vi "Panel.vi"(11 "Terminal in":refnum<class "Terminal.lvclass">) -> ()   [LabVIEW 2020, in "Terminal.lvlib" / "Terminal.lvclass"]
uses:
  Terminal.lvclass
  C:/Program Files (x86)/National Instruments/LabVIEW 2020/vi.lib/IlluminatedG/IG OOPanel/OOPanel/Panel/Panel.lvclass
  <vilib>/IlluminatedG/IG OOPanel/OOPanel/Panel/Basic UI State.ctl
  Terminal.lvclass/Terminal.ctl
  Key Event Data.ctl
  <vilib>/event_ctls.llb/eventvkey.ctl
  <vilib>/IlluminatedG/IG OOPanel/OOPanel/Panel/Panel.lvclass
  <vilib>/IlluminatedG/IG OOPanel/OOPanel/OOPanel.lvlib
  Terminal.lvlib
  C:/dev/IlluminatedG/lv-stream-terminal/Terminal/Terminal/Terminal.lvclass
panel:
  in  "Scrollbar":i32(c297)
  out "Overlay":picture
  out "Text":picture
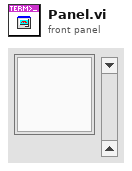
[diagram p1: front panel]
types:
  T1 = typedef "OOPanel.lvlib/Panel.lvclass/Basic UI State.ctl" = enum16{"Init", "Run", "Close"}
  T2 = typedef "Terminal.lvlib/Key Event Data.ctl" = cluster{"Char":i16, "VKey":T3, "ScanCode":i16, "Ctrl":bool}
  T3 = typedef "eventvkey.ctl" = enum16{"ASCII", "Enter", "Return", "Shift", "Ctrl", "Alt", "Cmd", "Opt", "Caps", "NumLock", "Clear", "Break", "Up", "Down", "Left", "Right", "Insert", "Delete", "Home", "End", "PageUp", "PageDown", "Escape", "Help", "Pause", "ScrollLock", "F1", "F2", "F3", "F4", "F5", "F6", "F7", "F8", "F9", "F10", "F11", "F12", "F13", "F14", "F15", "F16", "F17", "F18", "F19", "F20", "F21", "F22", "F23", "F24", "Play", "VolumeUp", "VolumeDown", "Mute", "Two Byte Char"}
  T4 = typedef "Terminal.lvlib/Terminal.lvclass/Incoming Events.ctl" = cluster{"Update":refnum<user-event>}
  T5 = typedef "OOPanel.lvlib/Panel.lvclass/Panel Events.ctl" = cluster{"Visbility":refnum<user-event>, "Close":refnum<user-event>}
  T6 = typedef "OOPanel.lvlib/Panel.lvclass/Visibility State.ctl" = enum16{"Idle", "Closed", "Hidden", "Visible", "Subpanel"}
  T7 = typedef "LVRectTypeDef.ctl" = cluster{"Left":i16, "Top":i16, "Right":i16, "Bottom":i16}
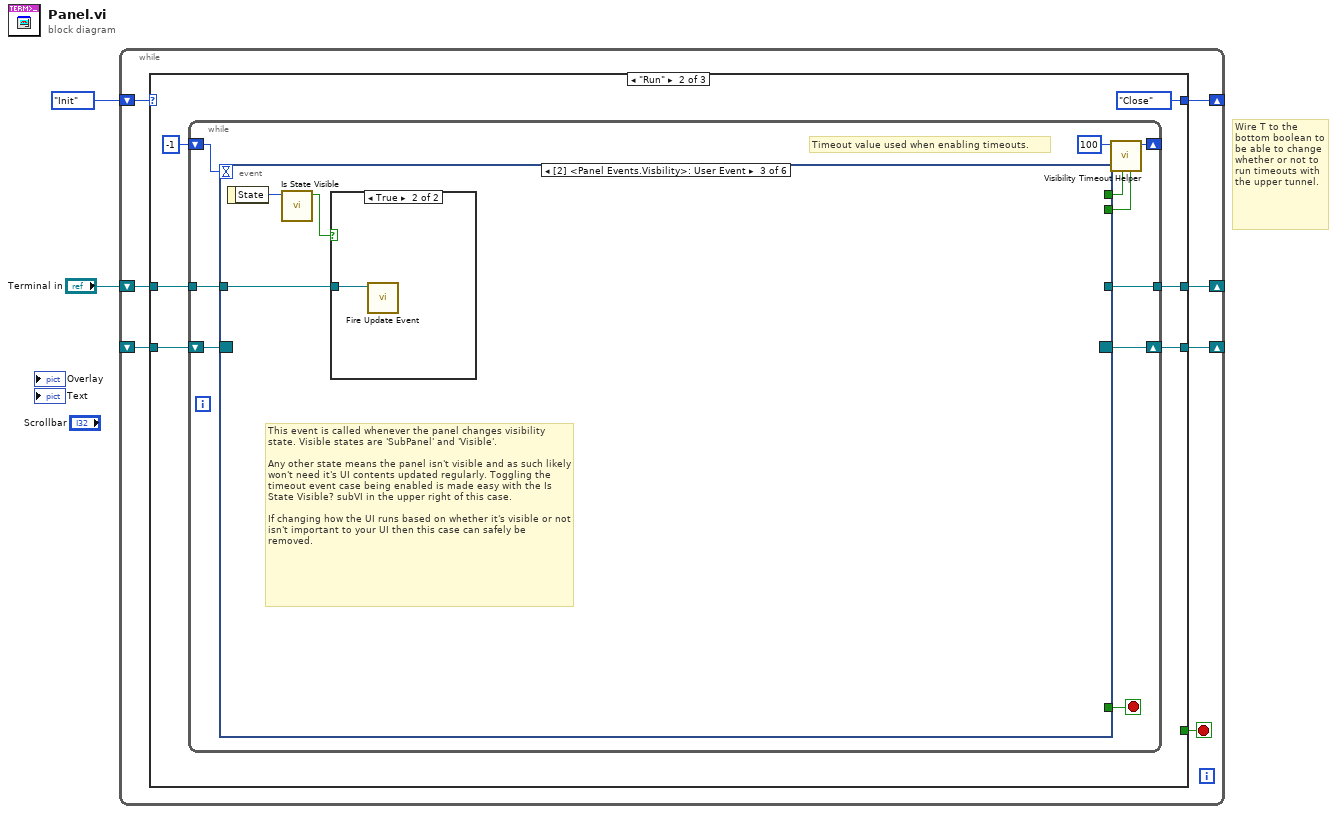
[diagram p0: block diagram]
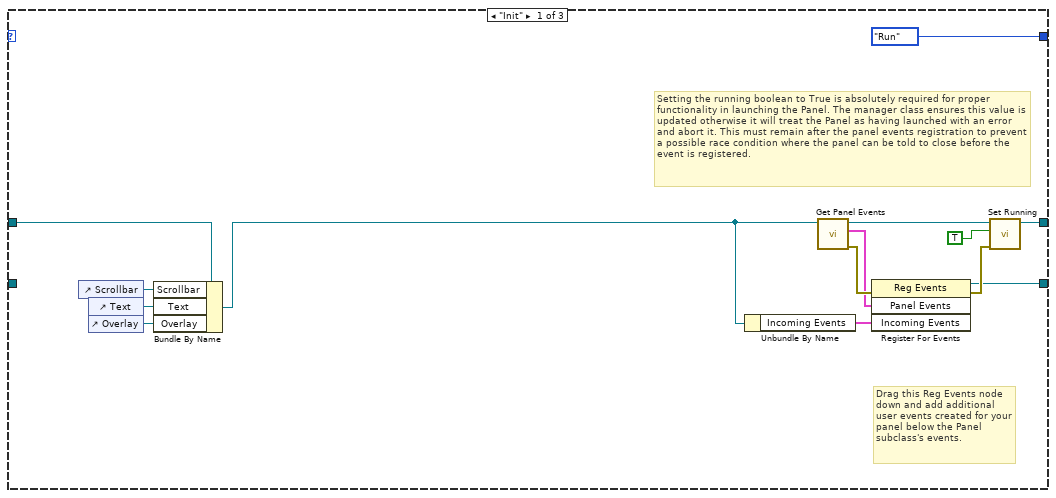
[diagram p2: hidden frame]
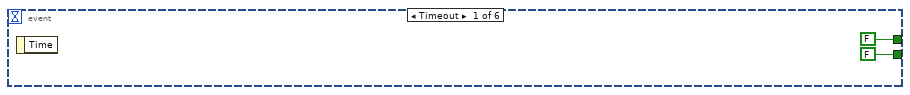
[diagram p3: hidden frame]
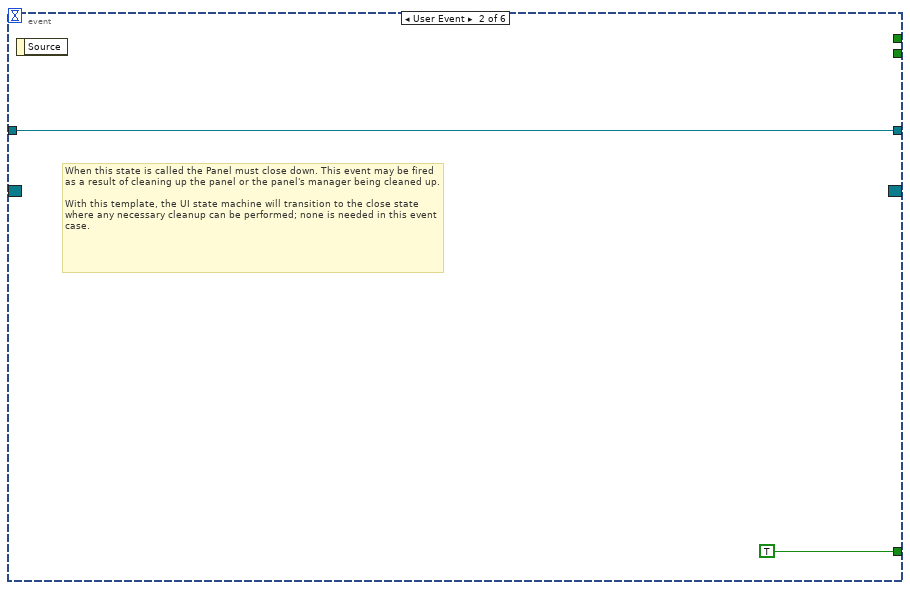
[diagram p4: hidden frame]
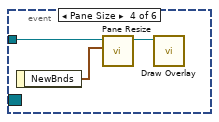
[diagram p6: hidden frame]
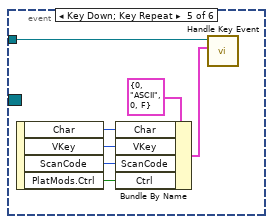
[diagram p7: hidden frame]
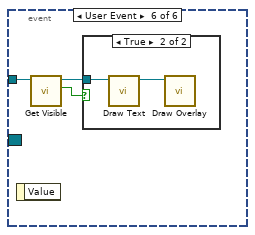
[diagram p8: hidden frame]
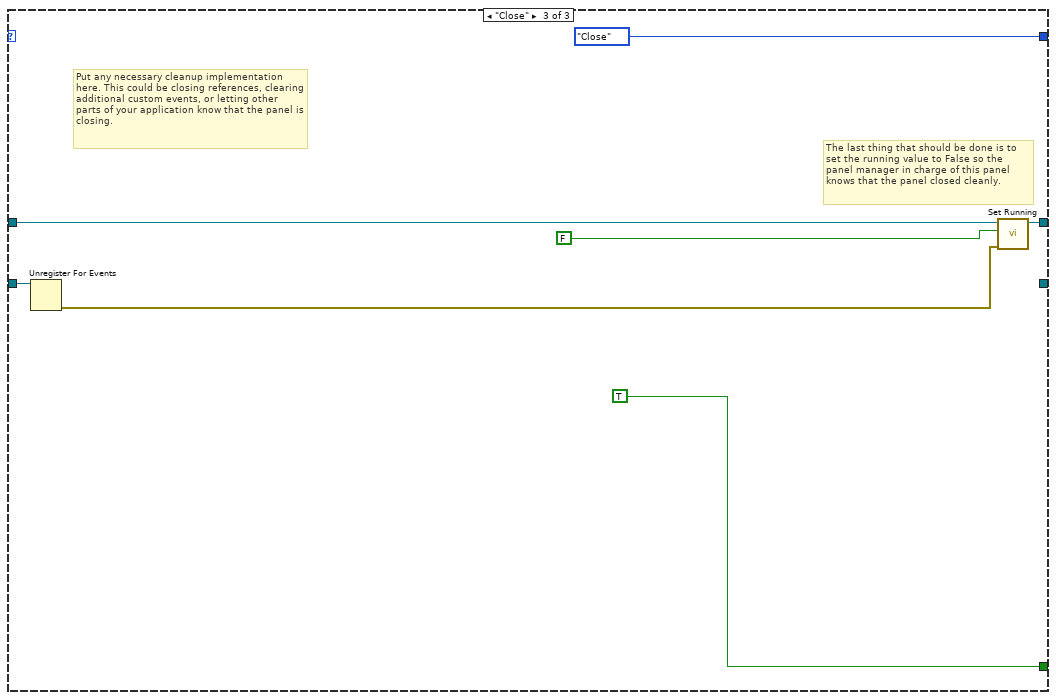
[diagram p10: hidden frame]
diagram:
  # "Wire T to the bottom boolean to be able to change whether or not to run timeouts with the upper tunnel."
  n1 = while {
    shift-right: [w8] -> _
    shift-left: _ -> [w9]
    shift-right: [w6] -> _
    shift-left: Basic_UI_State."Init" ("Basic UI State") -> [w7]
    shift-right: [w4] -> _
    shift-left: "Terminal in" -> [w3]
    stop <- w5 stop-if-true
    n2 = case shown="\"Run\"" w7 {
      tunnel: w9 -> [_ w29 w65]
      tunnel: [w17 w27 _] -> w8
      tunnel: [Basic_UI_State."Run" ("Basic UI State") Basic_UI_State."Close" ("Basic UI State") Basic_UI_State."Close" ("Basic UI State")] -> w6
      tunnel: [_ _ TRUE] -> w5
      tunnel: [w16 w24 w63] -> w4
      tunnel: w3 -> [w12 w25 w64]
      frame "Init" {
        # "Setting the running boolean to True is absolutely required for proper functionality in launching the Panel. The manager class ensures this value is updated otherwise it will treat the Panel as having launched with an error and abort it. This must remain after the panel events registration to prevent a possible race condition where the panel can be told to close before the event is registered."
        # "Drag this Reg Events node down and add additional user events created for your panel below the Panel subclass's events."
        n3 = control-ref of="Scrollbar"() -> (w15:refnum<vi>)
        n4 = control-ref of="Text"() -> (w14:refnum<vi>)
        n5 = control-ref of="Overlay"() -> (w13:refnum<vi>)
        n6 = Bundle By Name(cluster=w12, "Scrollbar"=w15, "Text"=w14, "Overlay"=w13) -> (w11:refnum<class "Terminal.lvclass">)
        n7 = Unbundle By Name(w11) -> ("Incoming Events"=w10:T4)
        n8 = call <vilib>:"Get Panel Events.vi"("Panel in"=w11) -> ("error out"=w23:errorcluster, "Panel Events"=w19:T5, "Panel out"=w20:refnum<class "Terminal.lvclass">)  [unwired: 8 in]
        n9 = register-events(error in=w23, w19, w10) -> (reference out=w17:refnum<event-registration>, error out=w21:errorcluster)  [unwired: 1 in]
        n10 = call <vilib>:"Set Running.vi"("error in (no error)"=w21, "Running"=TRUE, "Panel in"=w20) -> ("Panel out"=w16:refnum<class "Terminal.lvclass">)  [unwired: 7 in, 1 out]
      }
      frame "Run" {
        n11 = while {
          shift-right: [w35] -> w27
          shift-left: w29 -> [w36]
          shift-right: [w38] -> _
          shift-left: -1 ("Timeout") -> [w37]
          tunnel: w25 -> [w31]
          tunnel: [w30] -> w24
          stop <- w32 stop-if-true
          # "Timeout value used when enabling timeouts."
          n12 = event shown="[2] <Panel Events.Visbility>: User Event" {
            selector: w36 -> [_ _ _ _ _ _]
            dyn-events: [_ _ _ _ _ _] -> w35
            timeout: w37 -> [_ _ _ _ _ _]
            tunnel: [FALSE _ _ _ _ _] -> w34
            tunnel: [FALSE _ _ _ _ _] -> w33
            tunnel: [_ TRUE _ _ _ _] -> w32
            tunnel: w31 -> [_ w42 w44 w48 w52 w60]
            tunnel: [_ w42 _ _ _ _] -> w30
            event Timeout {
              n13 = event-data() -> ()  [unwired: 1 in, 1 out]
            }
            event User Event {
              # "When this state is called the Panel must close down. This event may be fired as a result of cleaning up the panel or the panel's manager being cleaned up.\n\nWith this template, the UI state machine will transition to the close state where any necessary cleanup can be performed; none is needed in this event case."
              n14 = event-data() -> ()  [unwired: 1 in, 1 out]
            }
            event User Event {
              # "This event is called whenever the panel changes visibility state. Visible states are 'SubPanel' and 'Visible'.\n\nAny other state means the panel isn't visible and as such likely won't need it's UI contents updated regularly. Toggling the timeout event case being enabled is made easy with the Is State Visible? subVI in the upper right of this case.\n\nIf changing how the UI runs based on whether it's visible or not isn't important to your UI then this case can safely be removed."
              n15 = event-data() -> ("State"=w46:T6)  [unwired: 1 in]
              n16 = call <vilib>:"Is State Visible.vi"("Visibility"=w46) -> ("Visible"=w45:bool)  [unwired: 10 in]
              n17 = case shown="True" w45 {
                tunnel: w44 -> [_ w47]
                frame False {
                }
                frame True {
                  n18 = call "Fire Update Event.vi"("Terminal in"=w47) -> ()  [unwired: 9 in, 2 out]
                }
              }
            }
            event Pane Size {
              n19 = event-data() -> ("NewBnds"=w50:T7)  [unwired: 1 in]
              n20 = call "Pane Resize.vi"("NewBnds"=w50, "Terminal in"=w48) -> ("Terminal out"=w49:refnum<class "Terminal.lvclass">)  [unwired: 8 in, 1 out]
              n21 = call "Draw Overlay.vi"("Terminal in"=w49) -> ()  [unwired: 9 in, 2 out]
            }
            event Key Down; Key Repeat {
              n22 = event-data() -> ("Char"=w56:i16, "VKey"=w55:T3, "ScanCode"=w54:i16, "PlatMods.Ctrl"=w53:bool)  [unwired: 1 in]
              n23 = Bundle By Name(cluster=T2 {"Char"=0, "VKey"=enum."ASCII", "ScanCode"=0, "Ctrl"=FALSE} ("Key Event Data"), "Char"=w56, "VKey"=w55, "ScanCode"=w54, "Ctrl"=w53) -> (w51:T2)
              n24 = call "Handle Key Event.vi"("Key Event Data"=w51, "Terminal in"=w52) -> ()  [unwired: 8 in, 2 out]
            }
            event User Event {
              n25 = event-data() -> ()  [unwired: 1 in, 1 out]
              n26 = call <vilib>:"Get Visible.vi"("Panel in"=w60) -> ("Visible"=w59:bool, "Panel out"=w58:refnum<class "Terminal.lvclass">)  [unwired: 8 in, 1 out]
              n27 = case shown="True" w59 {
                tunnel: w58 -> [_ w62]
                frame False {
                }
                frame True {
                  n28 = call "Draw Text.vi"("Terminal in"=w62) -> ("Terminal out"=w61:refnum<class "Terminal.lvclass">)  [unwired: 9 in, 1 out]
                  n29 = call "Draw Overlay.vi"("Terminal in"=w61) -> ()  [unwired: 9 in, 2 out]
                }
              }
            }
          }
          n30 = call <vilib>:"Visibility Timeout Helper.vi"("Update?"=w33, "Use Timeout?"=w34, "Visible Timeout mS"=100) -> ("Timeout"=w38:i32)  [unwired: 8 in]
        }
      }
      frame "Close" {
        # "Put any necessary cleanup implementation here. This could be closing references, clearing additional custom events, or letting other parts of your application know that the panel is closing."
        # "The last thing that should be done is to set the running value to False so the panel manager in charge of this panel knows that the panel closed cleanly."
        n31 = Unregister For Events(event registration refnum=w65) -> (error out=w67:errorcluster)  [unwired: 1 in]
        n32 = call <vilib>:"Set Running.vi"("error in (no error)"=w67, "Running"=FALSE, "Panel in"=w64) -> ("Panel out"=w63:refnum<class "Terminal.lvclass">)  [unwired: 7 in, 1 out]
      }
    }
  }
